vi "Read Fire (%).vi"(8 "error in (no error)":errorcluster, 11 "Cooker Actor in":refnum<class "Cooker Actor.lvclass">) -> (0 "error out":errorcluster, 2 "Fire (%)":dbl format="%.2f %%", 3 "Cooker Actor out":refnum<class "Cooker Actor.lvclass">)   [LabVIEW 2021, in "Cooker Actor.lvlib" / "Cooker Actor.lvclass"]
uses:
  Cooker Actor.lvclass
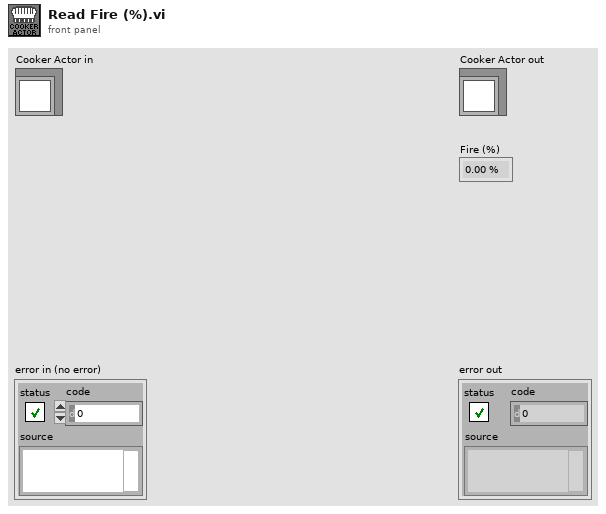
[diagram p1: front panel]
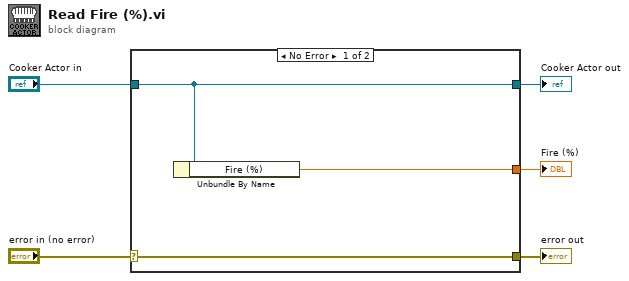
[diagram p0: block diagram]
diagram:
  n1 = case shown="No Error" "error in (no error)" {
    selector: "error in (no error)" -> [w8 w9]
    tunnel: [w8 w9] -> w4
    tunnel: [w7 w10] -> w2
    tunnel: "Cooker Actor in" -> [w7 w10]
    tunnel: [w6 _] -> w1
    frame No Error {
      n2 = Unbundle By Name(w7) -> ("Fire (%)"=w6:dbl)
    }
    frame Error {
    }
  }
  "error out" <- w4
  "Cooker Actor out" <- w2
  "Fire (%)" <- w1
